vi "basic_Check Voltage Current dt.vi"(8 "error in (no error)":errorcluster, 10 "current waveform":waveform(dbl), 11 "voltage waveform":waveform(dbl)) -> (0 "error out":errorcluster)   [LabVIEW 2013, in "NI_EP_Basic.lvlib"]
uses:
  <vilib>/addons/Electrical Power/Basic/NI_EP_Basic.lvlib
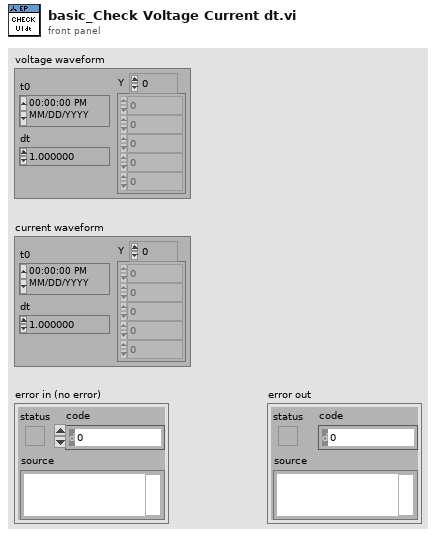
[diagram p1: front panel]
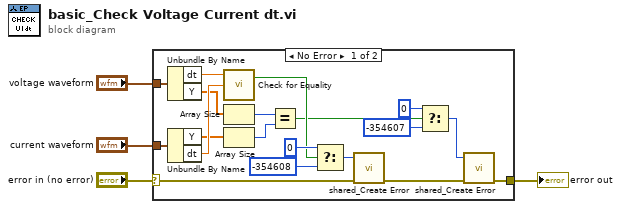
[diagram p0: block diagram]
diagram:
  n1 = case shown="No Error" "error in (no error)" {
    selector: "error in (no error)" -> [w21 w24]
    tunnel: "current waveform" -> [w22 _]
    tunnel: "voltage waveform" -> [w23 _]
    tunnel: [w5 w24] -> w1
    frame No Error {
      n2 = Unbundle By Name(w23) -> ("dt"=w17:dbl, "Y"=w13:dbl[])
      n3 = Unbundle By Name(w22) -> ("Y"=w14:dbl[], "dt"=w16:dbl)
      n4 = call <vilib>:"Check for Equality.vi"("n2"=w16, "n1"=w17) -> ("equal?"=w15:bool)  [unwired: 2 out]
      n5 = Array Size(array=w13) -> (size(s)=w12:i32)
      n6 = Array Size(array=w14) -> (size(s)=w11:i32)
      n7 = Equal?(x=w12, y=w11) -> (x = y?=w8:bool)
      n8 = Select(t=0, s=w15, f=-354608) -> (s? t:f=w20:i32)
      n9 = call <vilib>:"shared_Create Error.vi"("error in (no error)"=w21, "error code (0)"=w20) -> ("error out"=w6:errorcluster)  [unwired: 9 in]
      n10 = Select(t=0, s=w8, f=-354607) -> (s? t:f=w7:i32)
      n11 = call <vilib>:"shared_Create Error.vi"("error in (no error)"=w6, "error code (0)"=w7) -> ("error out"=w5:errorcluster)  [unwired: 9 in]
    }
    frame Error {
    }
  }
  "error out" <- w1
